vi "oauth2_authorize-pkce.vi"(6 "redirect_uri":string, 8 "error in (no error)":errorcluster, 9 "code_challenege_method":T1=enum."sha256", 10 "code_verifier":string, 11 "client_id":string) -> (0 "error out":errorcluster, 3 "auth_url":string)   [LabVIEW 2015, in "lv-dropbox.lvlib"]
uses:
  lv-dropbox.lvlib
  _controls/code_challenge_method.ctl
  private/cryptography/cryptography.lvlib
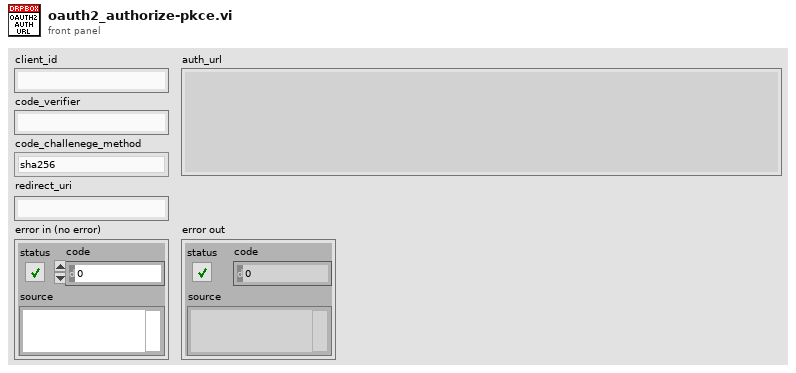
[diagram p1: front panel]
types:
  T1 = typedef "lv-dropbox.lvlib/code_challenge_method.ctl" = enum16{"<challenge_method>", "plain", "sha256"}
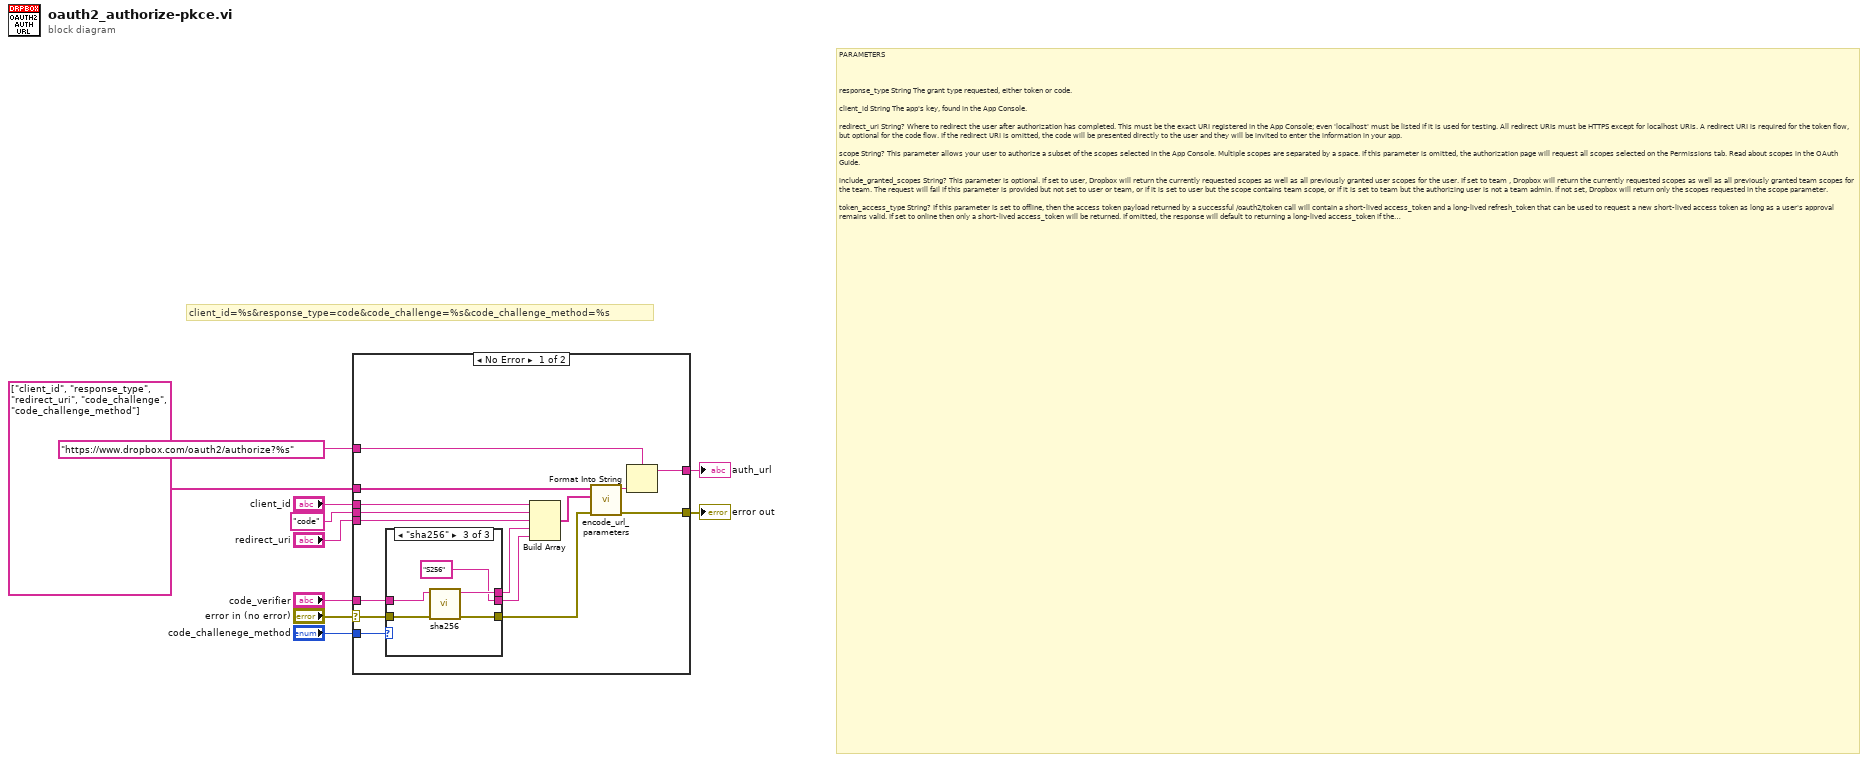
[diagram p0: block diagram]
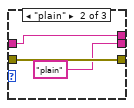
[diagram p3: hidden frame]
diagram:
  # "PARAMETERS\n\n\n\nresponse_type String The grant type requested, either token or code.\n\nclient_id String The app's key, found in the App Console.\n\nredirect_uri String? Where to redirect the user after authorization has completed. This must be the exact URI registered in the App Console; even 'localhost' must be listed if it is used for testing. All redirect URIs must be HTTPS except for localhost URIs. A redirect URI is required for the token flow, but optional for the code flow. If the redirect URI is omitted, the code will be presented directly to the user and they will be invited to enter the information in your app.\n\nscope String? This parameter allows your user to authorize a subset of the scopes selected in the App Console. Multiple scopes are separated by a space. If this parameter is omitted, the authorization page will request all scopes selected on the Permissions tab. Read about scopes in the OAuth Guide.\n\ninclude_granted_scopes String? This parameter is optional. If set to user, Dropbox will return the currently requested scopes as well as all previously granted user scopes for the user. If set to team , Dropbox will return the currently requested scopes as well as all previously granted team scopes for the team. The request will fail if this parameter is provided but not set to user or team, or if it is set to user but the scope contains team scope, or if it is set to team but the authorizing user is not a team admin. If not set, Dropbox will return only the scopes requested in the scope parameter.\n\ntoken_access_type String? If this parameter is set to offline, then the access token payload returned by a successful /oauth2/token call will contain a short-lived access_token and a long-lived refresh_token that can be used to request a new short-lived access token as long as a user's approval remains valid. If set to online then only a short-lived access_token will be returned. If omitted, the response will default to returning a long-lived access_token if they are allowed in the app console. If long-lived access tokens are disabled in the app console, this parameter defaults to online\n\nstate String? Up to 500 bytes of arbitrary data that will be passed back to your redirect URI. This parameter should be used to protect against cross-site request forgery (CSRF). See Sections 4.4.1.8 and 4.4.2.5 of the OAuth 2.0 threat model spec.\n\ncode_challenge String?(min_length=43, max_length=128) Part of the PKCE flow, the challenge should be an SHA-256 (S256) encoded value of a string that will serve as the code_verifier of the corresponding /oauth2/token call. Can can also be set to plain (plain).\n\ncode_challenge_method String? Defines the code challenge method. Can be set to S256 (recommended) or plain.\n\nrequire_role String? If this parameter is specified, the user will be asked to authorize with a particular type of Dropbox account, either work for a team account or personal for a personal account. Your app should still verify the type of Dropbox account after authorization since the user could modify or remove the require_role parameter.\n\nforce_reapprove Boolean? Whether or not to force the user to approve the app again if they've already done so. If false (default), a user who has already approved the application may be automatically redirected to the URI specified by redirect_uri. If true, the user will not be automatically redirected and will have to approve the app again.\n\ndisable_signup Boolean? When true (default is false) users will not be able to sign up for a Dropbox account via the authorization page. Instead, the authorization page will show a link to the Dropbox iOS app in the App Store. This is only intended for use when necessary for compliance with App Store policies.\n\nlocale String? If the locale specified is a supported language, Dropbox will direct users to a translated version of the authorization website. Locale tags should be IETF language tags.\n\nforce_reauthentication Boolean? When true (default is false) users will be signed out if they are currently signed in. This will make sure the user is brought to a page where they can create a new account or sign in to another account. This should only be used when there is a definite reason to believe that the user needs to sign in to a new or different account."
  # "client_id=%s&response_type=code&code_challenge=%s&code_challenge_method=%s"
  n1 = case shown="No Error" "error in (no error)" {
    selector: "error in (no error)" -> [w24 w35]
    tunnel: [w20 w35] -> w8
    tunnel: "https://www.dropbox.com/oauth2/authorize?%s" ("url") -> [w21 _]
    tunnel: "client_id" -> [w16 _]
    tunnel: "code_verifier" -> [w25 _]
    tunnel: [w23 _] -> w5
    tunnel: "code_challenege_method" -> [w22 _]
    tunnel: string[] ["client_id", "response_type", "redirect_uri", "code_challenge", "code_challenge_method"] -> [w17 _]
    tunnel: "code" -> [w14 _]
    tunnel: "redirect_uri" -> [w13 _]
    frame No Error {
      n2 = case shown="\"sha256\"" w22 {
        tunnel: [_ w29 w34] -> w12
        tunnel: w25 -> [_ w29 w33]
        tunnel: w24 -> [w26 w28 w32]
        tunnel: [w26 w28 w31] -> w19
        tunnel: [_ "plain" ("url") "S256" ("url")] -> w11
        frame Default {
        }
        frame "plain" {
        }
        frame "sha256" {
          n3 = call "sha256.vi"("error in (no error)"=w32, "data_decoded"=w33) -> ("error out"=w31:errorcluster, "data_encoded"=w34:string)  [unwired: 8 in]
        }
      }
      n4 = Build Array(w16, w14, w13, w12, w11) -> (w15:string[])
      n5 = call "encode_url_parameters.vi"("error in (no error)"=w19, "value []"=w15, "key []"=w17) -> ("error out"=w20:errorcluster, "url_encoded_string"=w18:string)  [unwired: 7 in]
      n6 = Format Into String(format string=w21, w18) -> (resulting string=w23:string)  [unwired: 2 in, 1 out]
    }
    frame Error {
    }
  }
  "error out" <- w8
  "auth_url" <- w5
